vi "Get a_n.vi"(10 "n":i32, 11 "Analytical Serial Arm Class in":refnum<class "NI_Robotics_Analytical Serial Arm Class.lvclass">) -> (2 "a_n":dbl, 3 "Analytical Serial Arm Class out":refnum<class "NI_Robotics_Analytical Serial Arm Class.lvclass">)   [LabVIEW 2017, in "NI_Robotics_Analytical Serial Arm Class.lvclass"]
uses:
  <vilib>/robotics/Kinematics/Analytical/Generic/NI_Robotics_Analytical Serial Arm Class.lvclass
  c:/Program Files (x86)/National Instruments/LabVIEW 2017/vi.lib/robotics/Kinematics/Robot/NI_Robotics_Serial Robot Arm.lvclass
  <vilib>/robotics/Kinematics/Link/NI_Robotics_Link.lvclass/NI_Robotics_Link.ctl
  <vilib>/robotics/Kinematics/Analytical/Generic/Accessors/Read a_n0.vi
  <vilib>/robotics/Kinematics/Robot/NI_Robotics_Serial Robot Arm.lvclass
  <vilib>/robotics/Kinematics/Link/NI_Robotics_Link.lvclass
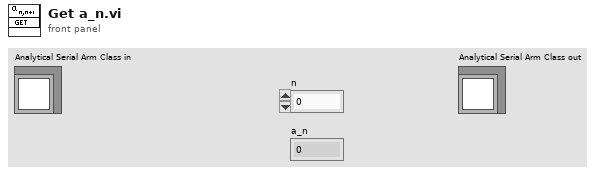
[diagram p1: front panel]
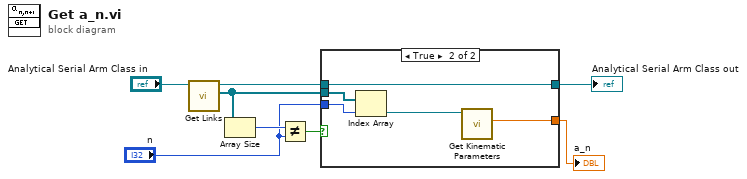
[diagram p0: block diagram]
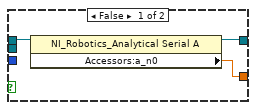
[diagram p2: hidden frame]
diagram:
  n1 = call <vilib>:"Get Links.vi"("serial arm in"="Analytical Serial Arm Class in") -> ("links"=w6:refnum<class "NI_Robotics_Link.lvclass">[], "serial arm out"=w2:refnum<class "NI_Robotics_Analytical Serial Arm Class.lvclass">)  [unwired: 8 in, 1 out]
  n2 = Array Size(array=w6) -> (size(s)=w5:i32)
  n3 = Not Equal?(x=w5, y="n") -> (x != y?=w3:bool)
  n4 = case shown="True" w3 {
    tunnel: "n" -> [_ w16]
    tunnel: w6 -> [_ w14]
    tunnel: [w9 w13] -> w7
    tunnel: w2 -> [w11 w12]
    tunnel: [w10 w12] -> w1
    frame False {
      n5 = property class="NI_Robotics_Analytical Serial A"(reference=w11) -> (reference out=w10:refnum<class "NI_Robotics_Analytical Serial Arm Class.lvclass">, "Accessors:a_n0"=w9:dbl)  [unwired: 1 in, 1 out]
    }
    frame True {
      n6 = Index Array(array=w14, index=w16) -> (element=w15:refnum<class "NI_Robotics_Link.lvclass">)
      n7 = call <vilib>:"Get Kinematic Parameters.vi"("NI_Robotics_Link in"=w15) -> ("Length"=w13:dbl)  [unwired: 6 in, 4 out]
    }
  }
  "Analytical Serial Arm Class out" <- w1
  "a_n" <- w7
